vi "oa_Check for Even-Angle Position Continuity.vi"(7 "reset in":bool, 8 "error in (no error)":errorcluster, 9 "even-angle position info":T1) -> (0 "error out":errorcluster, 1 "even-angle position info dup":T1, 5 "position not continuous":bool)   [LabVIEW 2017]
uses:
  <vilib>/addons/Sound and Vibration/Order Analysis/Misc/OAT Position Info.ctl
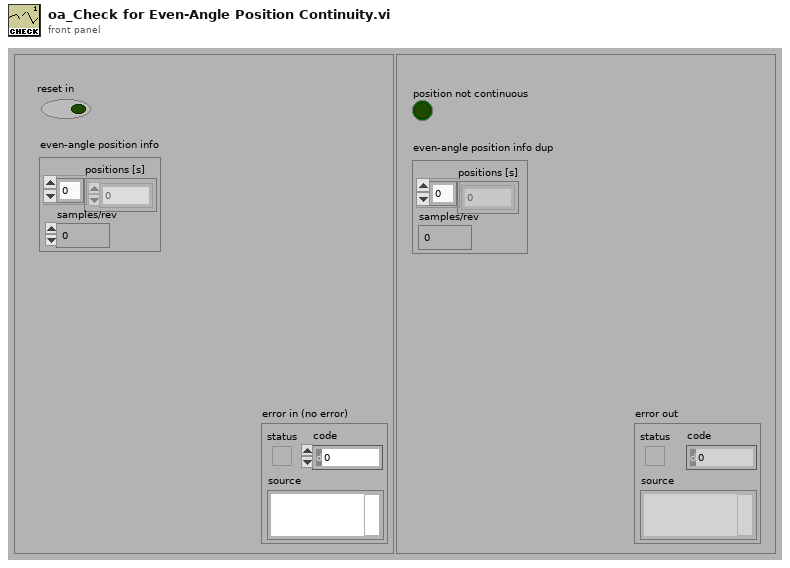
[diagram p1: front panel]
types:
  T1 = typedef "OAT Position Info.ctl" = cluster{"positions [s]":dbl[], "samples/rev":dbl}
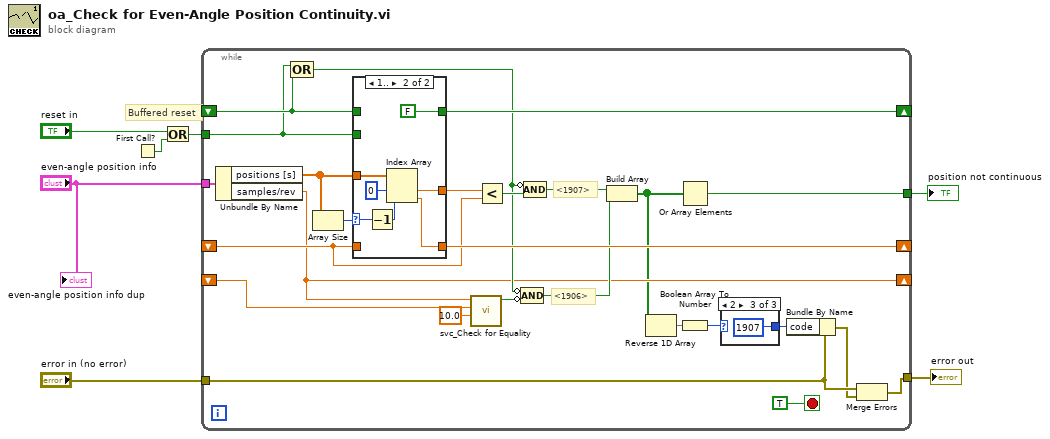
[diagram p0: block diagram]
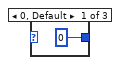
[diagram p2: hidden frame]
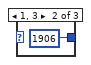
[diagram p3: hidden frame]
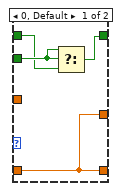
[diagram p4: hidden frame]
diagram:
  # "Buffered reset"
  n1 = First Call?() -> (First Call?: T/F=w5:bool)
  n2 = Or(x="reset in", y=w5) -> (x .or. y?=w3:bool)
  n3 = while {
    tunnel: "error in (no error)" -> [w12]
    shift-right: [w29] -> _
    shift-left: _ -> [w26]
    tunnel: "even-angle position info" -> [w32]
    shift-right: [w19] -> _
    shift-left: _ -> [w18]
    shift-right: [w28] -> _
    shift-left: _ -> [w25]
    tunnel: w3 -> [w24]
    tunnel: [w10] -> w2
    tunnel: [w8] -> w1
    stop <- TRUE stop-if-true
    # "<1906>"
    # "<1907>"
    n4 = Unbundle By Name(w32) -> ("positions [s]"=w30:dbl[], "samples/rev"=w19:dbl)
    n5 = Compound Arithmetic op=OR(w24, w25) -> (w22:bool)
    n6 = Array Size(array=w30) -> (size(s)=w31:i32)
    n7 = case shown="1.." w31 {
      selector: w31 -> [_ w45]
      tunnel: w30 -> [_ w47]
      tunnel: [w40 w43] -> w29
      tunnel: [w40 w42] -> w27
      tunnel: w26 -> [w40 _]
      tunnel: w24 -> [w39 _]
      tunnel: w25 -> [w38 _]
      tunnel: [w37 FALSE] -> w28
      frame 0, Default {
        n8 = Select(t=w39, s=w39, f=w38) -> (s? t:f=w37:bool)
      }
      frame 1.. {
        n9 = Decrement(x=w45) -> (x-1=w44:i32)
        n10 = Index Array(array=w47, index #1=0 ("index"), index #2=w44) -> (element #1=w42:dbl, element #2=w43:dbl)
      }
    }
    n11 = call <vilib>:"svc_Check for Equality.vi"("desired precision"=10.0, "n2"=w18, "n1"=w19) -> ("equal?"=w16:bool)  [unwired: 7 in, 1 out]
    n12 = Less?(x=w27, y=w26) -> (x < y?=w23:bool)
    n13 = Compound Arithmetic op=AND(invert w22, invert w16) -> (w20:bool)
    n14 = Compound Arithmetic op=AND(invert w22, w23) -> (w21:bool)
    n15 = Build Array(w21, w20) -> (w9:bool[])
    n16 = Reverse 1D Array(array=w9) -> (reversed array=w15:bool[])
    n17 = Or Array Elements(Boolean array=w9) -> (logical OR=w8:bool)
    n18 = Boolean Array To Number(Boolean array=w15) -> (number=w14:u32)
    n19 = case shown="2" w14 {
      tunnel: [0 ("code") 1906 ("code") 1907 ("code")] -> w13
      frame 0, Default {
      }
      frame 1, 3 {
      }
      frame 2 {
      }
    }
    n20 = Bundle By Name(cluster=w12, "code"=w13) -> (w11:errorcluster)
    n21 = Merge Errors(w12, w11) -> (w10:errorcluster)
  }
  "error out" <- w2
  "position not continuous" <- w1
  "even-angle position info dup" <- "even-angle position info"
